vi "Write success.vi"(8 "error in (no error)":errorcluster, 10 "success":bool, 11 "mqttCmd in":refnum<class "mqttCmd.lvclass">) -> (0 "error out":errorcluster, 3 "mqttCmd out":refnum<class "mqttCmd.lvclass">)   [LabVIEW 2020, in "mqttCmd.lvclass"]
uses:
  mqttCmd.lvclass
  mqttCmd.lvclass/mqttCmd.ctl
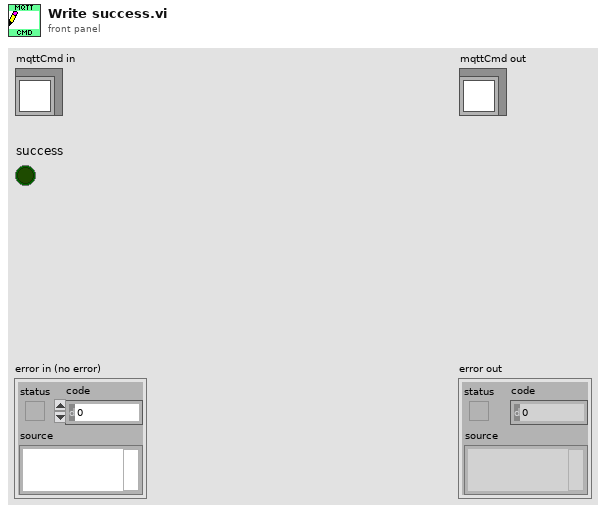
[diagram p1: front panel]
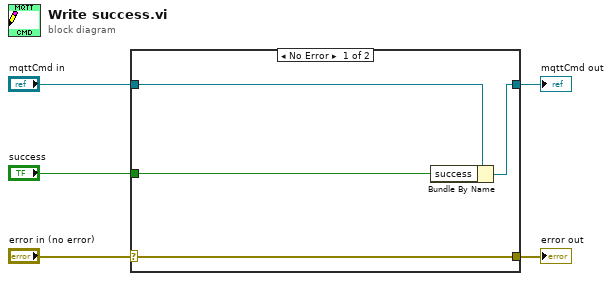
[diagram p0: block diagram]
diagram:
  n1 = case shown="No Error" "error in (no error)" {
    selector: "error in (no error)" -> [w9 w10]
    tunnel: [w9 w10] -> w4
    tunnel: [w7 w11] -> w2
    tunnel: "mqttCmd in" -> [w8 w11]
    tunnel: "success" -> [w6 _]
    frame No Error {
      n2 = Bundle By Name(cluster=w8, "success"=w6) -> (w7:refnum<class "mqttCmd.lvclass">)
    }
    frame Error {
    }
  }
  "error out" <- w4
  "mqttCmd out" <- w2
